vi "GPS Ublox M8N.vi"() -> (0 "Error Out":errorcluster)   [LabVIEW 2021, in "NMEA_GPS Ublox M8N.lvlib"]
uses:
  NMEA_GPS Ublox M8N.lvlib
  NMEA/NMEA_GNVTG Data.ctl
  NMEA/NMEA_Mode.ctl
  NMEA/NMEA_GNRMC Data.ctl
  NMEA/NMEA_Latitude Direction.ctl
  NMEA/NMEA_Longitude Direction.ctl
  NMEA/NMEA_GNGGA Data.ctl
  NMEA/NMEA_GPS Quality.ctl
  NMEA/NMEA_Type.ctl
  D:/My Projects/GitHub/3. GMap 1.7.0/Data/GMap.NET.WindowsForms.dll
  Data/GMap.NET.WindowsForms.dll
  Map Functions/ctlSeqFNs.ctl
  Map Functions/ctlInput4PtsColl.ctl
  fbf526f2-a788-4282-be0c-3f4d0c04ab2b.vi
  6f17bc59-fa4d-4478-9a37-96364ebc542e.vi
  Map Functions/Global Var.vi
  <vilib>/Instr/_visa.llb/VISA Configure Serial Port (Instr).vi
  <vilib>/Utility/file.llb/Write Delimited Spreadsheet (string).vi
  D:/My Projects/GitHub/3. GMap 1.7.0/Data/GMap.NET.Core.dll
  Data/GMap.NET.Core.dll
panel:
  out "MouseLng":dbl caption="Lng" format="%#.6f"
  out "MouseLat":dbl caption="Lat" format="%#.6f"
  in  "Mode":T1(ring)=enum."ServerAndCache"
  in  "Map Providers":string(combo)="27"
  in  "Zoom":dbl(slide)=14.0 min=1.0 max=20.0 step=1.0 scale=0.0..20.0
  in  "Zoom & Center":bool caption="btnZoom & Center"
  in  "Add Marker":bool
  out "Map Error":errorcluster
  in  "Error In 2":errorcluster
  in  "Marker Tooltip":enum16{"On Mouse Move", "Never", "Always"}(ring)=enum."Always"
  in  "Marker ToolTip":string="You Are Here..."
  in  "dotNetGMap":refnum<k24>(container)
  in  "Stop":bool
  in  "Serial Settings":T2={"Baud Rate"=38400, "Data Bits"=8, "Parity"=enum."None", "Stop Bits"=10, "Flow Control"=0} {"Flow Control" items=["None"=0, "XON/XOFF"=1, "RTS/CTS"=2, "DTR/DSR"=4]; "Stop Bits" items=["1.0"=10, "1.5"=15, "2.0"=20]; "Data Bits" min=5 max=8 step=1; "Baud Rate" items=["75"=75, "110"=110, "134"=134, "150"=150, "300"=300, "600"=600, "1200"=1200, "1800"=1800, "2400"=2400, "4800"=4800, "7200"=7200, "9600"=9600, "14400"=14400, "19200"=19200, "28800"=28800, "38400"=38400, "56000"=56000, "57600"=57600, "115200"=115200, "128000"=128000, "230400"=230400]}
  out "Read Data":string
  in  "COM Port":refnum<visa-resource-name>="COM18"
  in  "Timeout (ms)":u32=10000
  in  "End read on Termination Character?":bool=TRUE
  in  "Termination Char (0xA = '\\n' = LF)":u8=10 format="%.0x"
  in  "XON Character":u8=17 format="%.0x"
  in  "XOFF Character":u8=19 format="%.0x"
  in  "Input Buffer Size":u32=4096
  in  "Bytes to Read":u32=1000
  out "Actual Bytes Read":u32
  out "MessageType":T3
  in  "Error In":errorcluster
  out "$GNGGA Message":T4={"TimeStamp"=timestamp(0 s since 1904-01-01), "Latitude"=0.0, "Latitude Direction"=enum."", "Longitude"=1.0, "Longitude Direction"=enum."", "GPS Quality"=enum."GPS fix (SPS)", "Number of Satellites"=0, "Horizontal Dilution of Precision"=0.0, "Altitude above Mean-Sea-Level"=0.0, "Geoidal Separation"=0.0, "Time Since Last DGPS Update"=0.0, "DGPS Reference Station ID"=0} {"Time Since Last DGPS Update" format="%.02f [s]"; "Geoidal Separation" format="%.02f [m]"; "Altitude above Mean-Sea-Level" format="%.02f [m]"; "Horizontal Dilution of Precision" format="%.02f [HDOP]"; "Longitude" format="%0.4f [long]"; "Latitude" format="%.04f [lat]"; "TimeStamp" format="%<%.2X>T"}
  out "Latitude":dbl format="%.6f"
  out "Longitude":dbl format="%.6f"
  out "Data":string[][](table)
  out "$GNRMC Message":T8={"TimeStamp"=timestamp(0 s since 1904-01-01), "Validity"=FALSE, "Latitude"=0.0, "Latitude Direction"=enum."North", "Longitude"=0.0, "Longitude Direction"=enum."East", "Speed in Knots"=0.0, "True Course"=0.0, "Date Stamp"=timestamp(0 s since 1904-01-01), "Magnetic Variation (East/West)"=0.0} {"Magnetic Variation (East/West)" format="%.02f [deg]"; "Date Stamp" format="%<%x>T"; "True Course" format="%.02f [deg]"; "Speed in Knots" format="%.02f [kts]"; "Longitude" format="%0.4f [long]"; "Latitude" format="%.04f [lat]"; "TimeStamp" format="%<%.2X>T"}
  out "$GNVTG Message":T9={"True Course over Ground"=0.0, "Magnetic Course over Ground"=0.0, "Speed over Ground in knots"=0.0, "Speed over Ground in km/h"=1.0, "Mode"=""} {"Speed over Ground in km/h" format="%.02f [km/h]"; "Speed over Ground in knots" format="%.02f [kts]"; "Magnetic Course over Ground" format="%.02f [deg]"; "True Course over Ground" format="%.02f [deg]"}
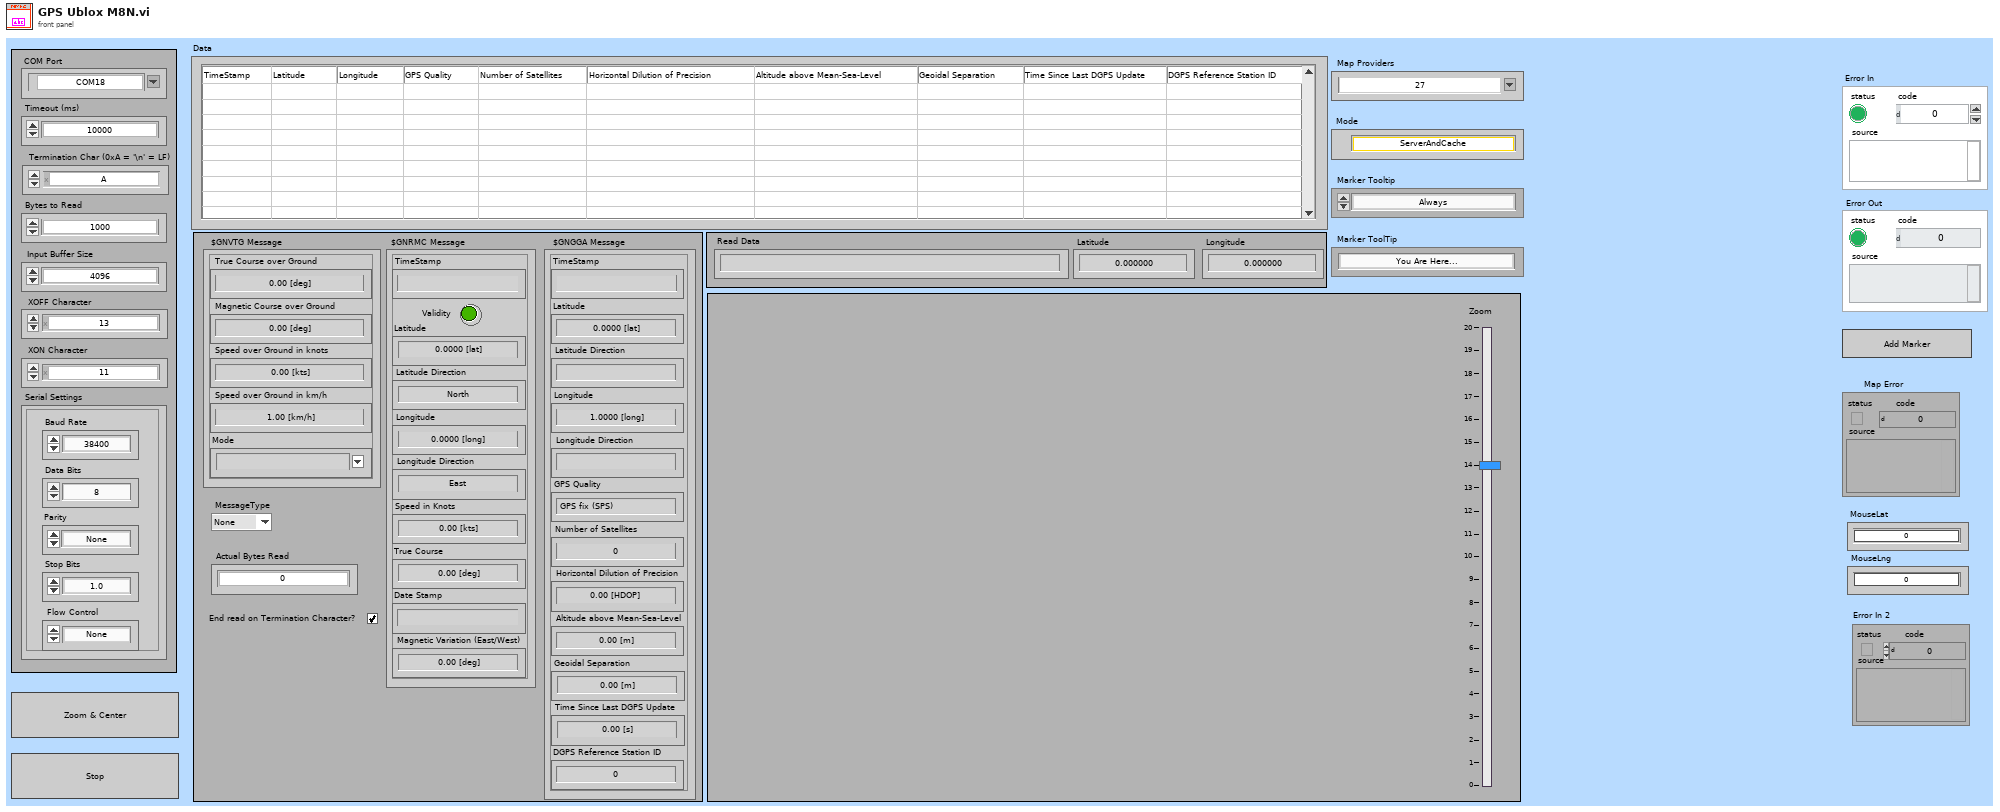
[diagram p1: front panel]
types:
  T1 = enum16{"ServerOnly", "ServerAndCache", "CacheOnly"}
  T2 = cluster{"Baud Rate":u32, "Data Bits":u16, "Parity":enum16{"None", "Odd", "Even", "Mark", "Space"}, "Stop Bits":u16, "Flow Control":u16}
  T3 = typedef "NMEA_GPS Ublox M8N.lvlib/NMEA_Type.ctl" = enum16{"None", "GGA", "VTG", "RMC"}
  T4 = typedef "NMEA_GPS Ublox M8N.lvlib/NMEA_GNGGA Data.ctl" = cluster{"TimeStamp":timestamp, "Latitude":dbl, "Latitude Direction":T5, "Longitude":dbl, "Longitude Direction":T6, "GPS Quality":T7, "Number of Satellites":i32, "Horizontal Dilution of Precision":dbl, "Altitude above Mean-Sea-Level":dbl, "Geoidal Separation":dbl, "Time Since Last DGPS Update":dbl, "DGPS Reference Station ID":i32}
  T5 = typedef "NMEA_GPS Ublox M8N.lvlib/NMEA_Latitude Direction.ctl" = enum16{"", "North", "South"}
  T6 = typedef "NMEA_GPS Ublox M8N.lvlib/NMEA_Longitude Direction.ctl" = enum16{"", "East", "West"}
  T7 = typedef "NMEA_GPS Ublox M8N.lvlib/NMEA_GPS Quality.ctl" = enum16{"Invalid", "GPS fix (SPS)", "DGPS fix", "PPS fix", "Real Time Kinematic", "Float RTK", "estimated", "Manual input mode", "Simulation mode"}
  T8 = typedef "NMEA_GPS Ublox M8N.lvlib/NMEA_GNRMC Data.ctl" = cluster{"TimeStamp":timestamp, "Validity":bool, "Latitude":dbl, "Latitude Direction":T5, "Longitude":dbl, "Longitude Direction":T6, "Speed in Knots":dbl, "True Course":dbl, "Date Stamp":timestamp, "Magnetic Variation (East/West)":dbl}
  T9 = typedef "NMEA_GPS Ublox M8N.lvlib/NMEA_GNVTG Data.ctl" = cluster{"True Course over Ground":dbl, "Magnetic Course over Ground":dbl, "Speed over Ground in knots":dbl, "Speed over Ground in km/h":dbl, "Mode":T10}
  T10 = typedef "NMEA_GPS Ublox M8N.lvlib/NMEA_Mode.ctl" = string
  T11 = typedef "NMEA_GPS Ublox M8N.lvlib/ctlSeqFNs.ctl" = enum16{"Pre - Initialize 0", "Pre - Initialize 1", "Pre - Initialize 2", "Pre - Initialize 3", "Idle", "Set Provider", "Set Scale", "Add Overlay", "Points - Create List (Container)", "Map - Marker Add Or Rmv", "Map - Markers Autofit", "Map - Markers Clear", "Error", "Exit"}
  T12 = enum32{"Invalid", "Standard", "Closed", "Hidden", "Minimized", "Maximized"}
  T13 = cluster{"Idx|Addr|City|Prov|Lng|Lat|Checked":string[], "tbCtlGUI":refnum<vi>, "PinDropLatDblClck":refnum<vi>, "PinDropLngDblClck":refnum<vi>, "MouseLat":refnum<vi>, "MouseLng":refnum<vi>, "RefScale":refnum<vi>, "RefcmbProviders":refnum<vi>, "RefMode":refnum<vi>, "EvntRefGMap":refnum<k27>, "arrRefProviders":refnum<k24>[], "arrProviderNms":string[], "dotNetGMap":refnum<k24>, "PathCurr":path, "VIRef":refnum<vi>, "arrOverlayNames":string[], "arrOverlayRefs":refnum<k24>[], "RefPointsCollPoly":refnum<k24>, "arrLatLngDF":dbl[][][], "arrLatLngPoly":dbl[][], "arrPointKeyWordOrID":string[], "MouseLatDblClck":refnum<vi>, "MouseLngDblClck":refnum<vi>}
  T14 = typedef "NMEA_GPS Ublox M8N.lvlib/ctlInput4PtsColl.ctl" = cluster{"arrLatLngActv":dbl[][], "ptKeyorID":string[], "Add":bool}
  T15 = enum16{"none", "arrow", "blue", "blue_small", "blue_dot", "blue_pushpin", "brown_small", "gray_small", "green", "green_small", "green_dot", "green_pushpin", "green_big_go", "yellow", "yellow_small", "yellow_dot", "yellow_big_pause", "yellow_pushpin", "lightblue", "lightblue_dot", "lightblue_pushpin", "orange", "orange_small", "orange_dot", "pink", "pink_dot", "pink_pushpin", "purple", "purple_small", "purple_dot", "purple_pushpin", "red", "red_small", "red_dot", "red_pushpin", "red_big_stop", "black_small", "white_small"}
  T16 = cluster{"arrOverlayRefs":refnum<k24>[], "RefPointsColl in":refnum<k24>, "arrPointKeyWordOrID":string[], "PtLatLn+KywrdOrID":T14, "arrLatLngActv":dbl[][]}
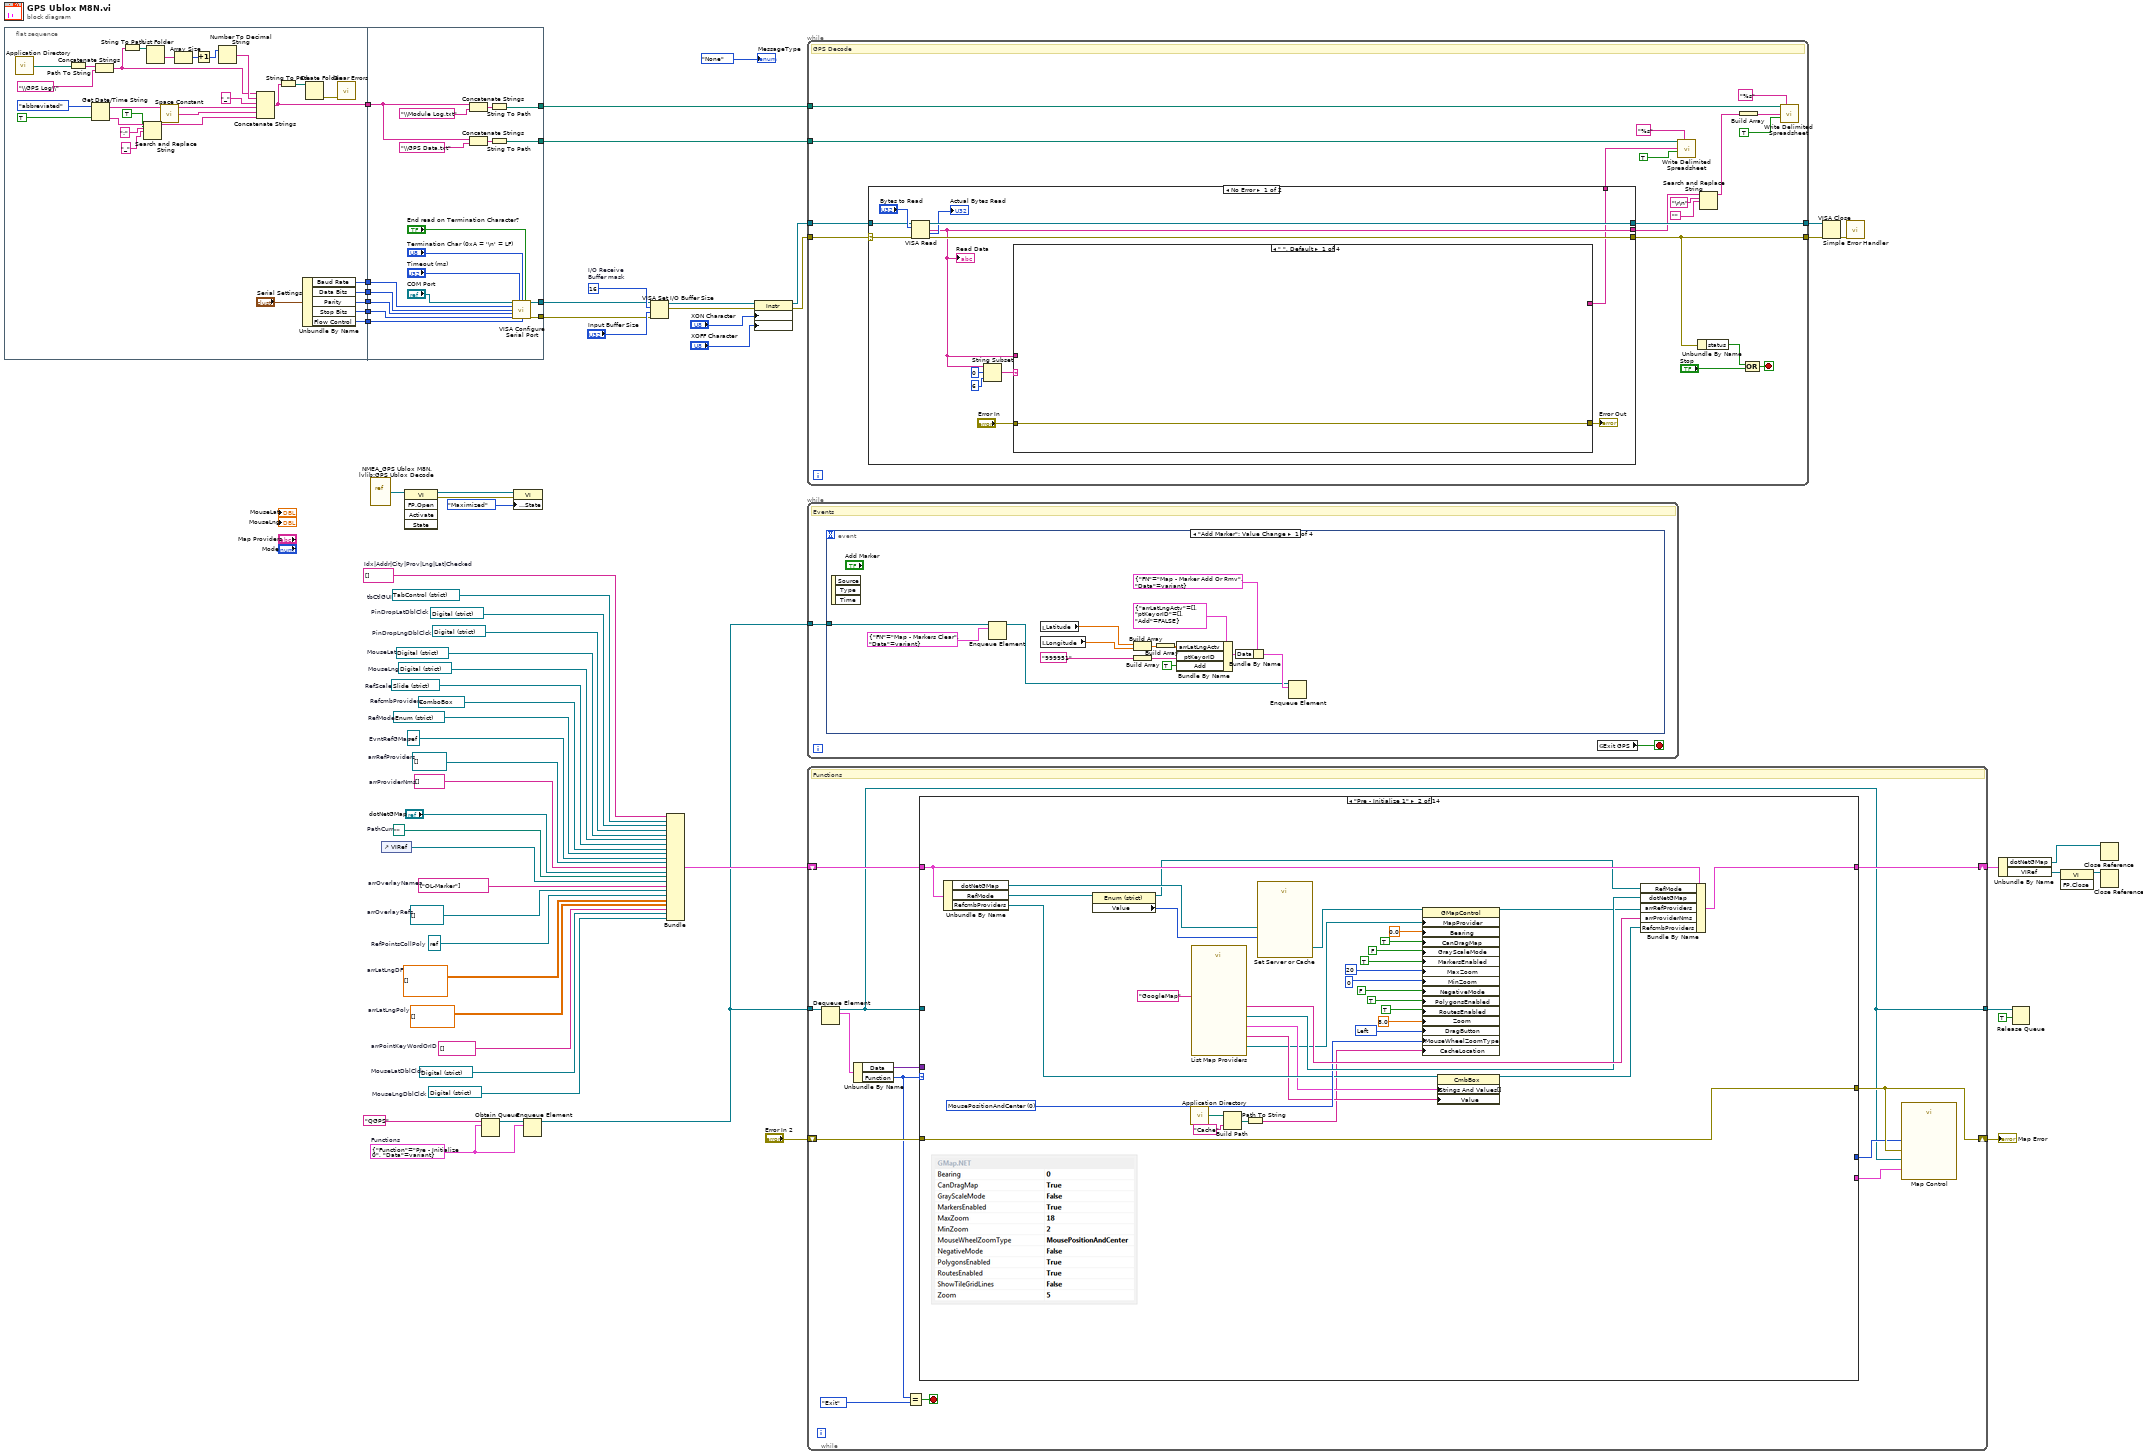
[diagram p0: block diagram]
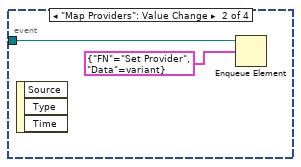
[diagram p2: hidden frame]
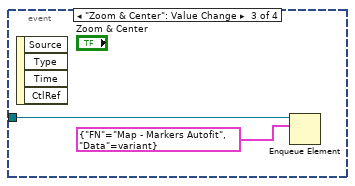
[diagram p3: hidden frame]
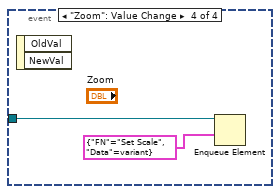
[diagram p4: hidden frame]
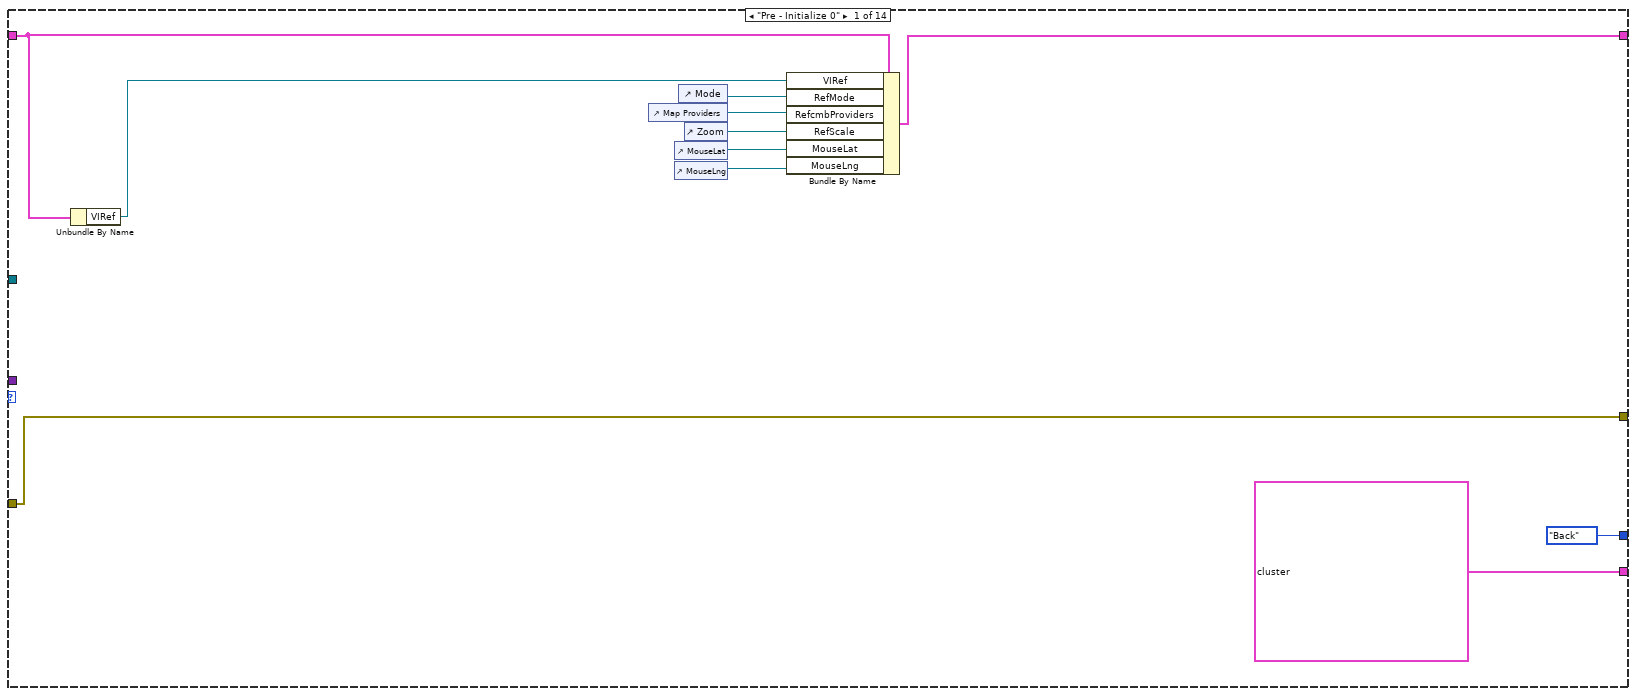
[diagram p5: hidden frame]
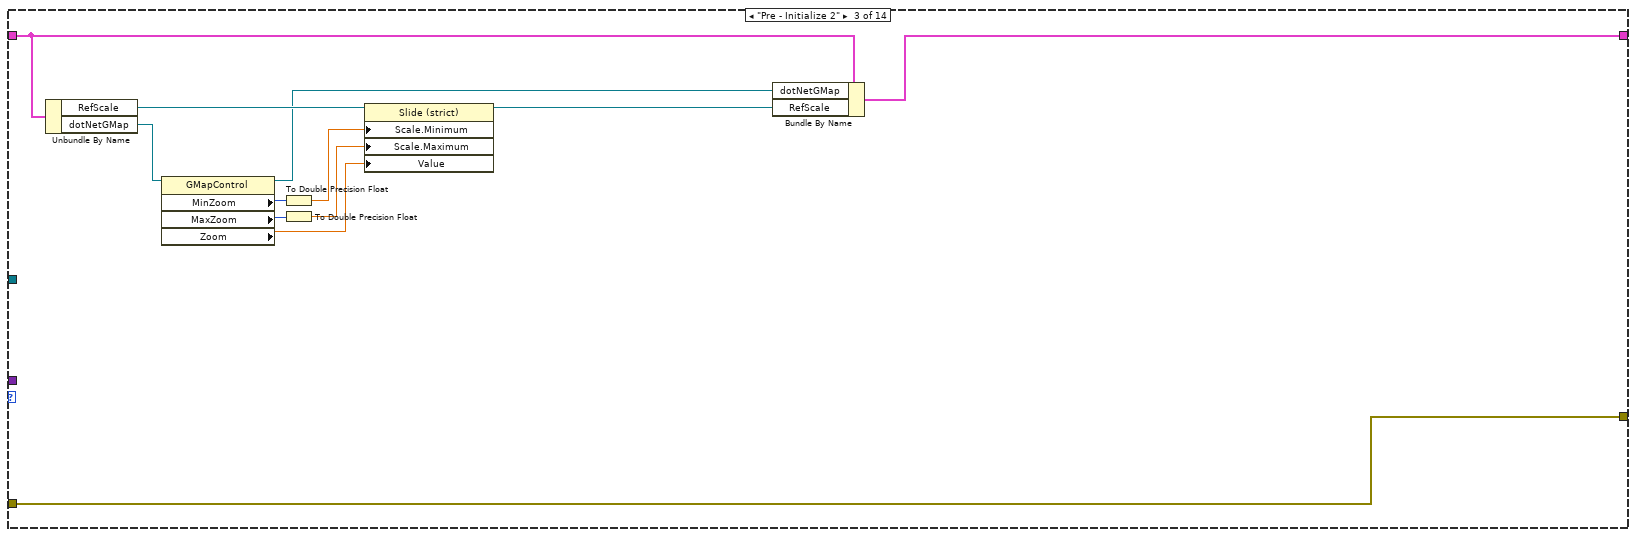
[diagram p6: hidden frame]
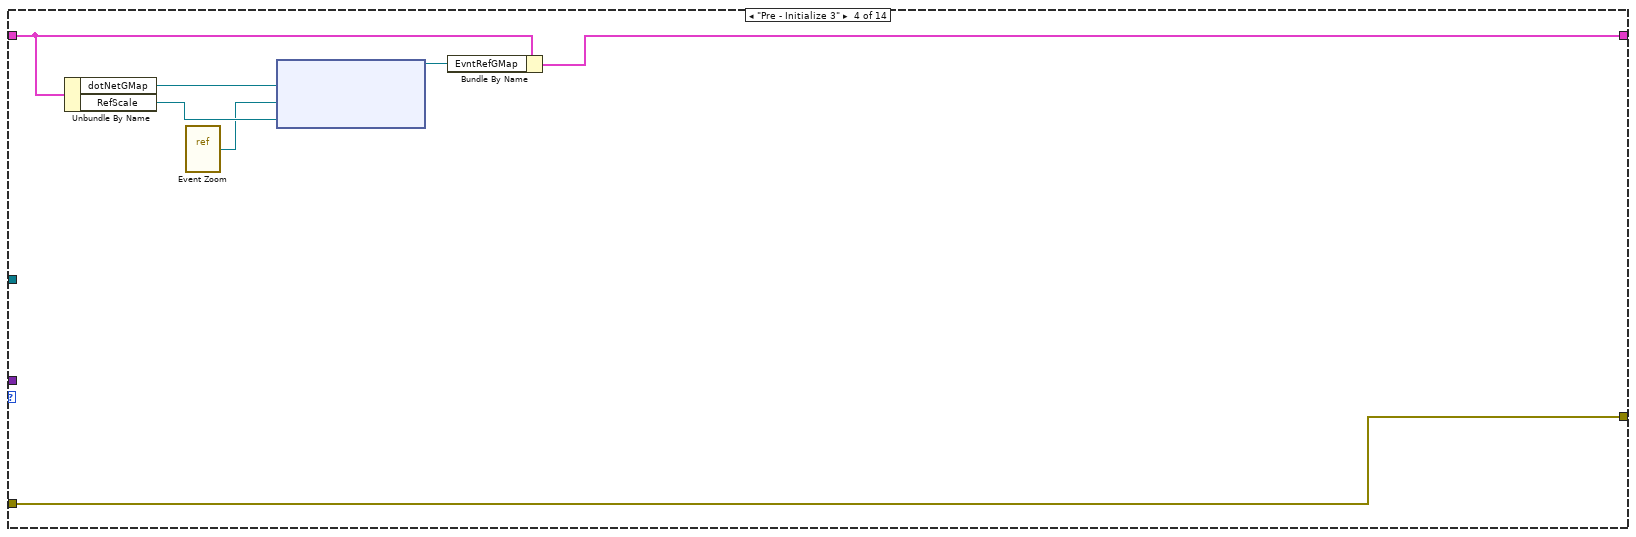
[diagram p7: hidden frame]
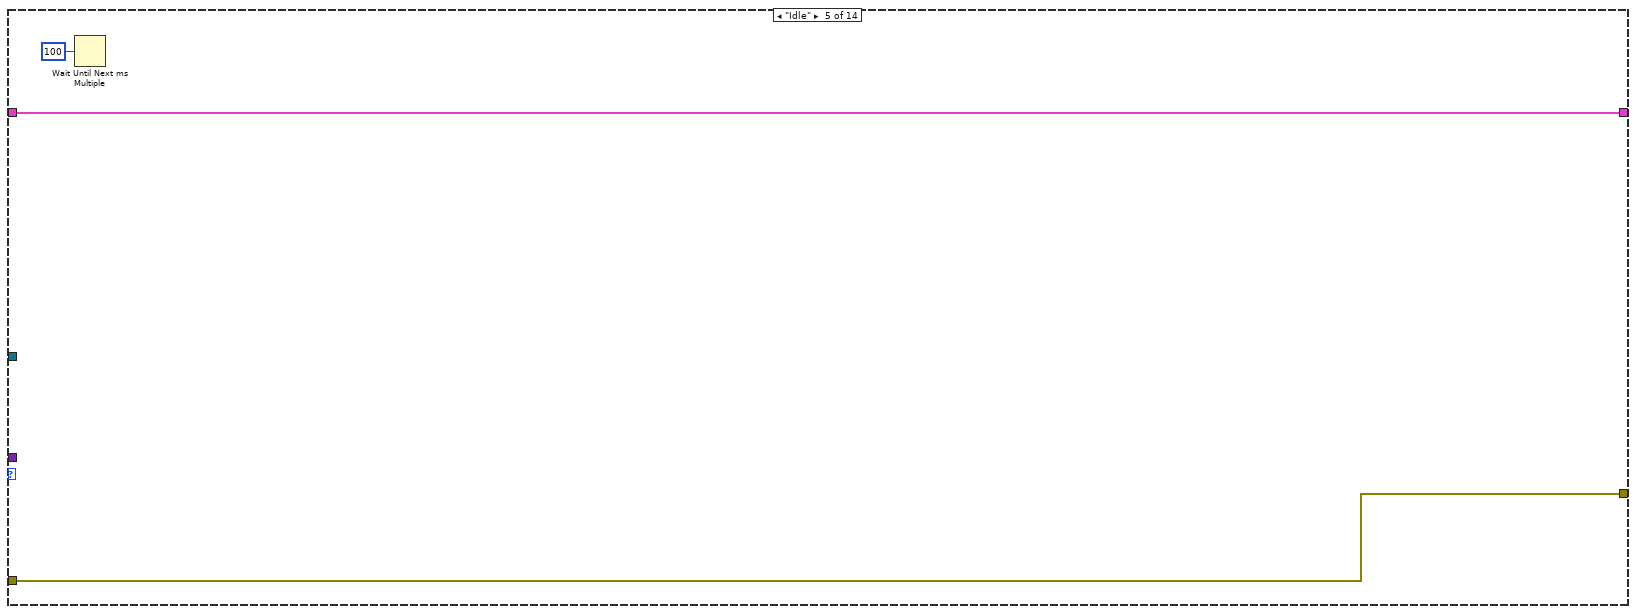
[diagram p8: hidden frame]
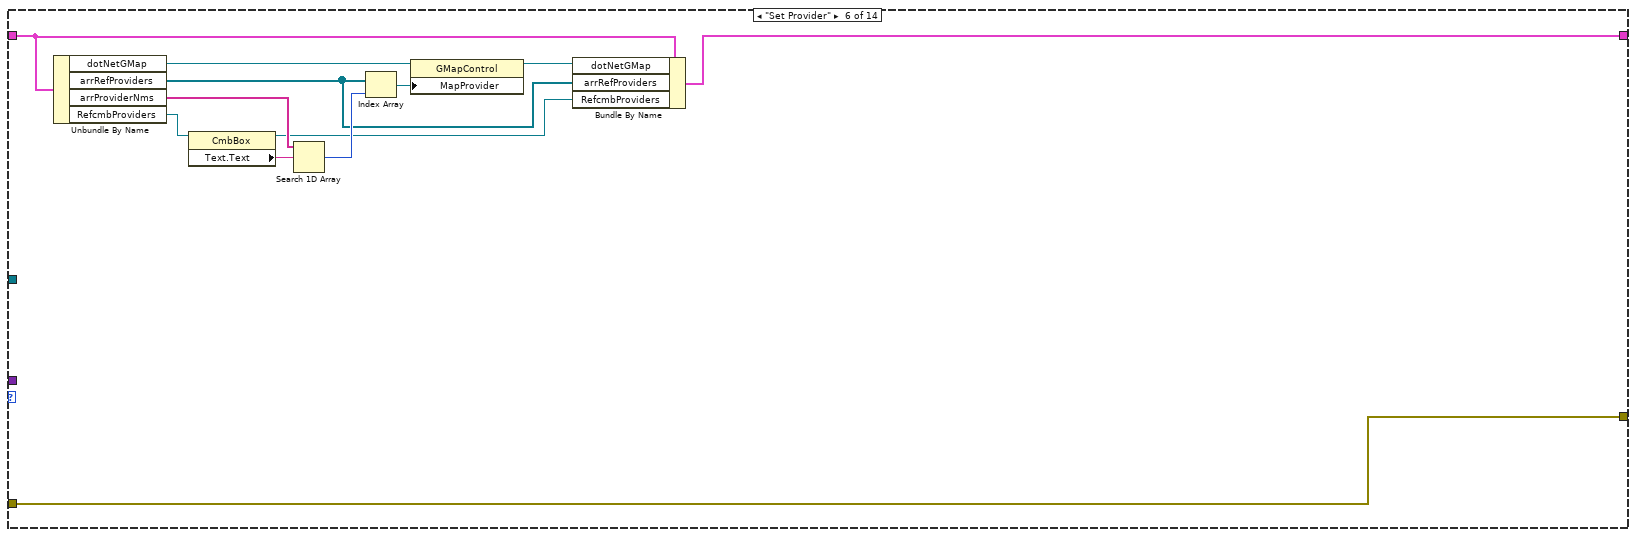
[diagram p9: hidden frame]
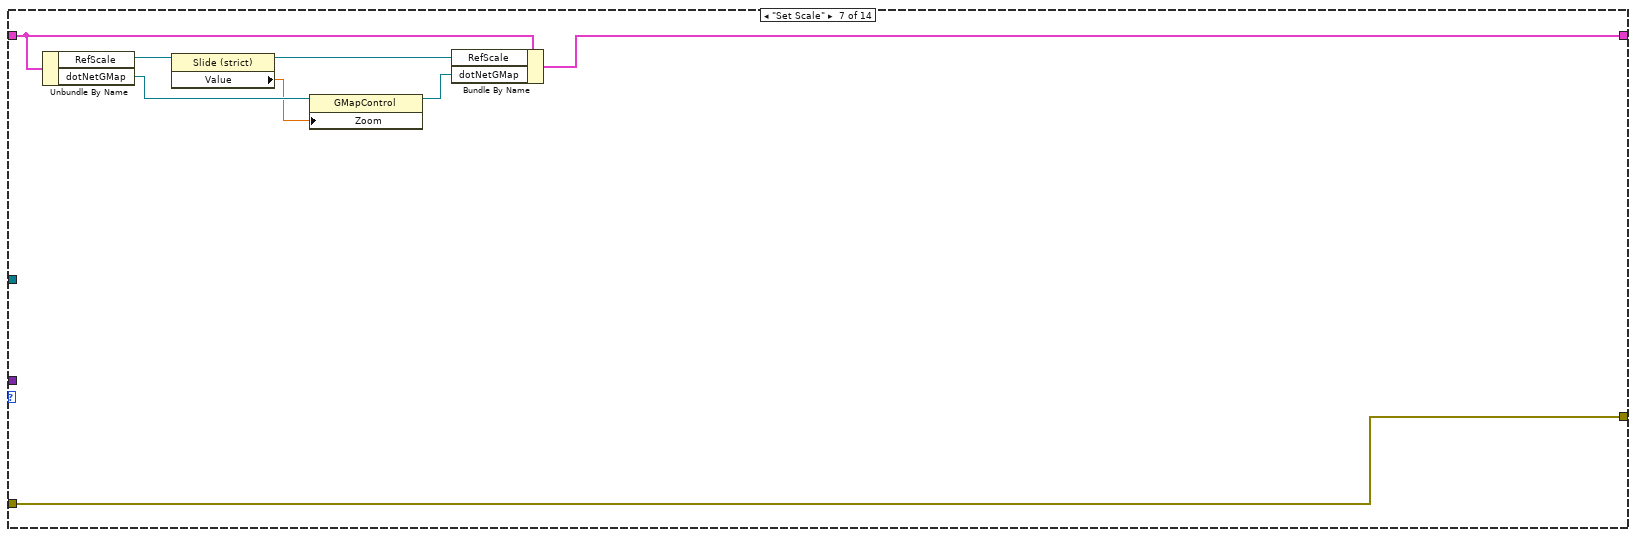
[diagram p10: hidden frame]
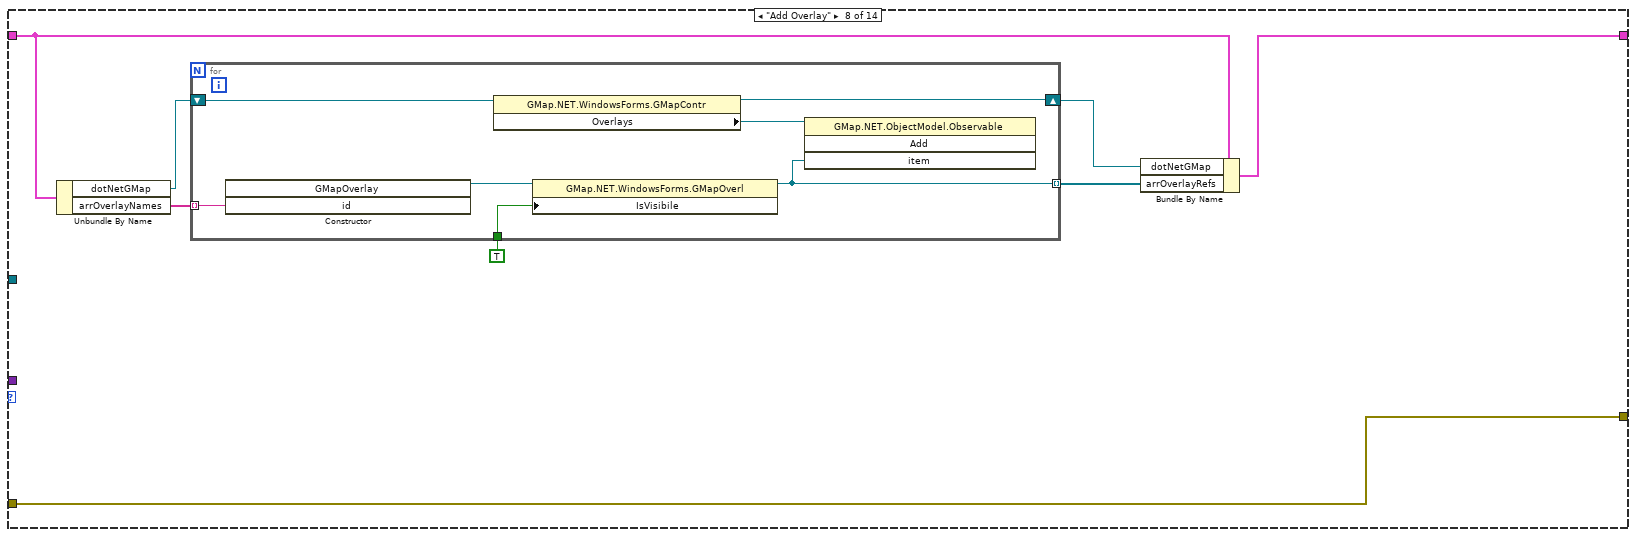
[diagram p11: hidden frame]
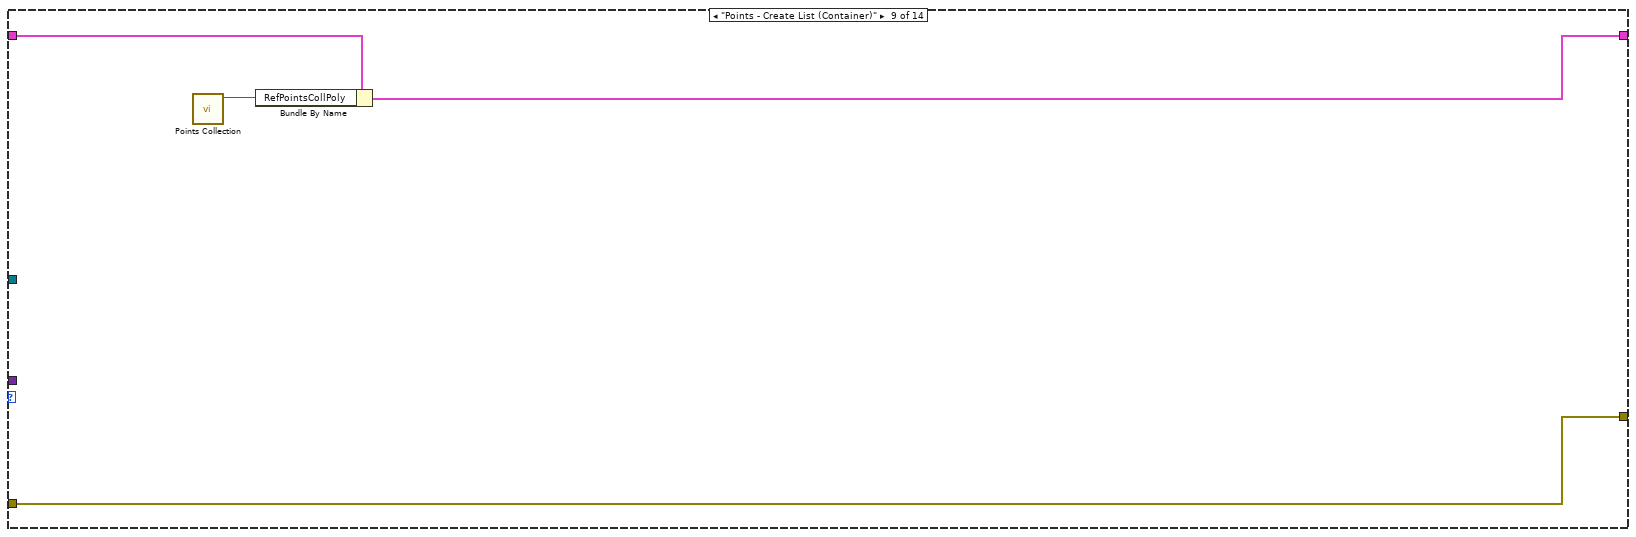
[diagram p12: hidden frame]
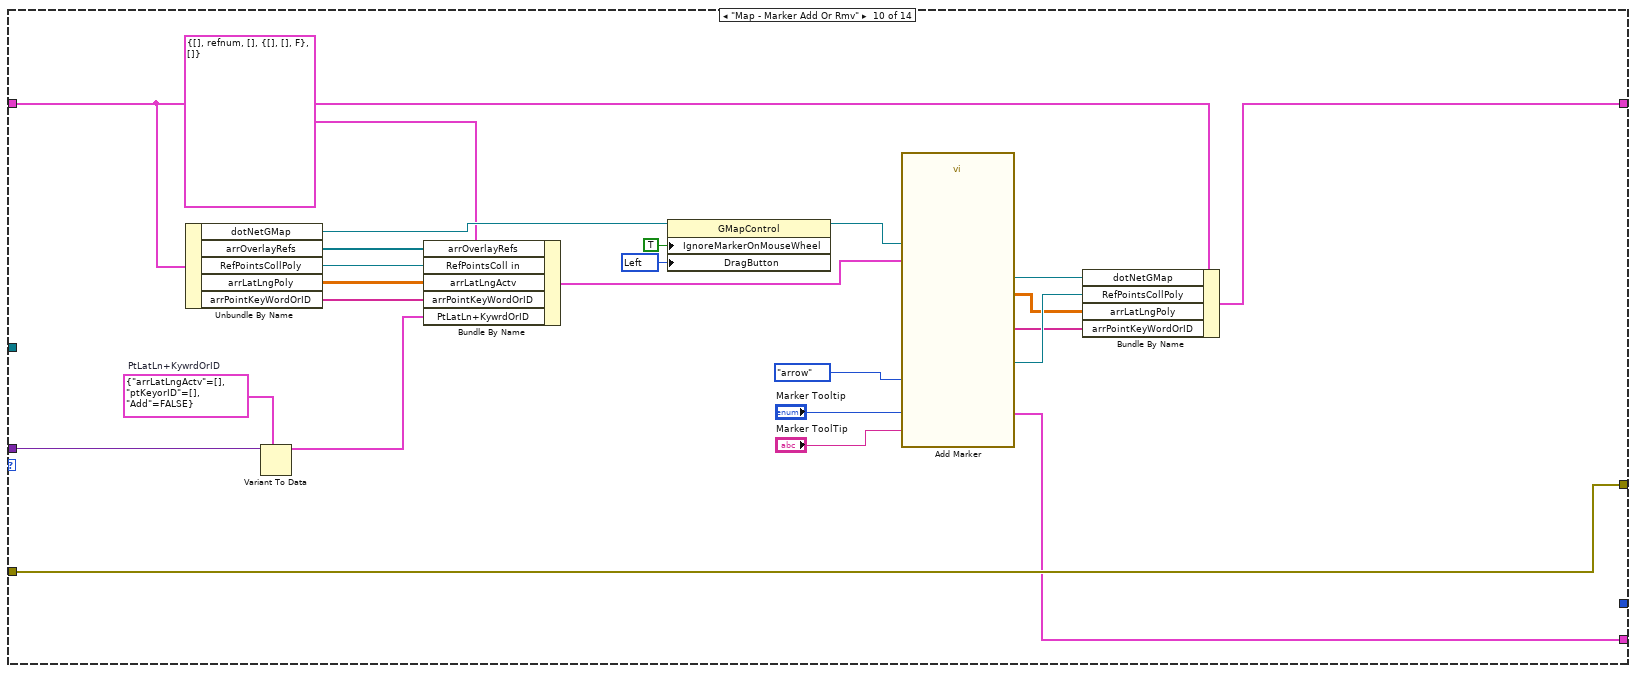
[diagram p13: hidden frame]
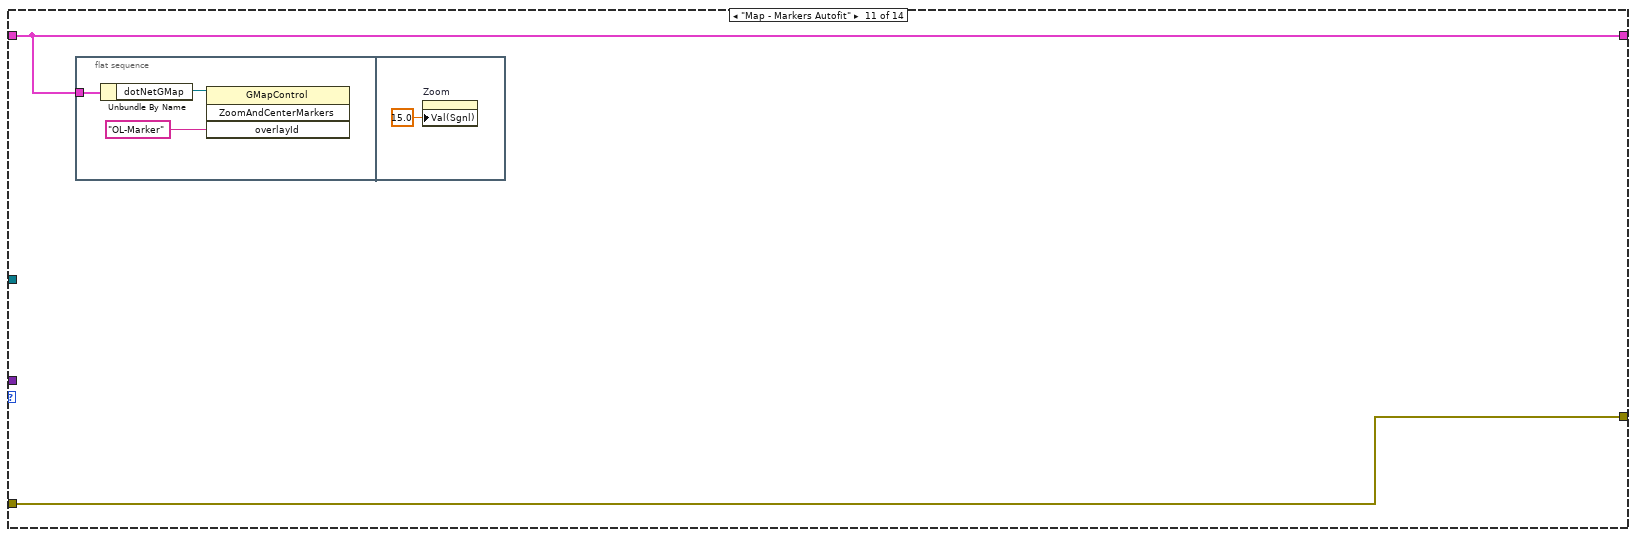
[diagram p14: hidden frame]
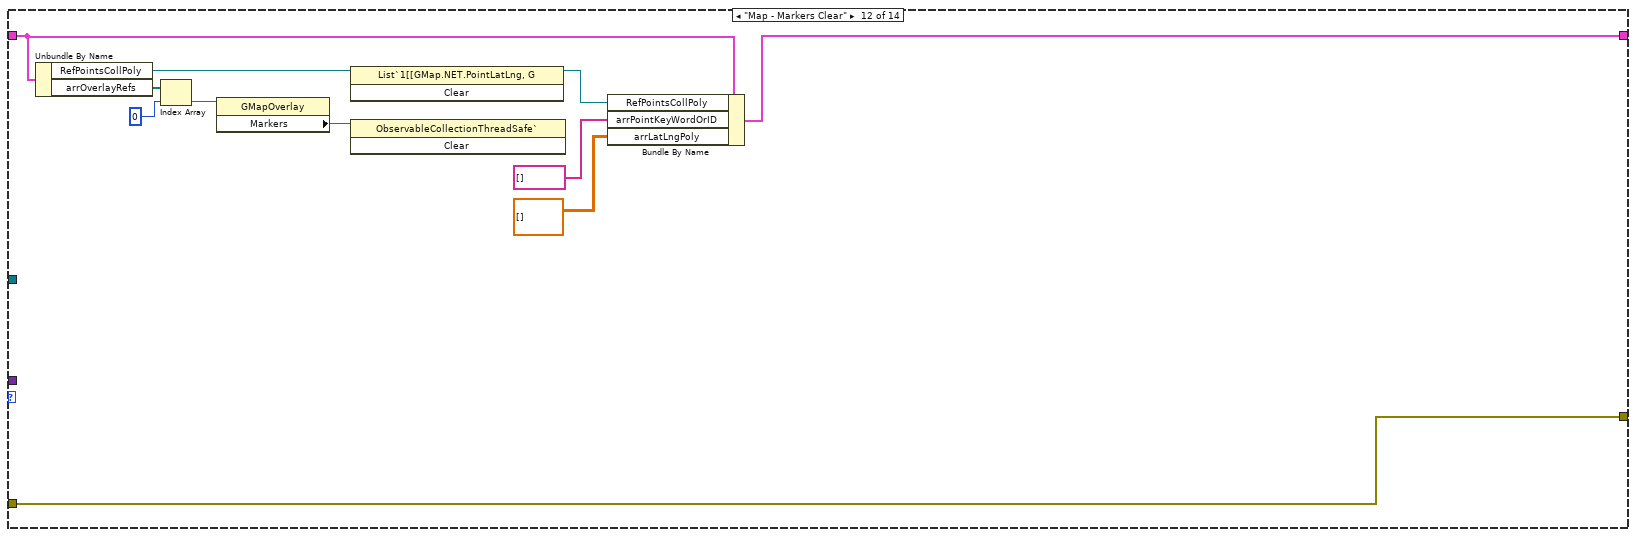
[diagram p15: hidden frame]
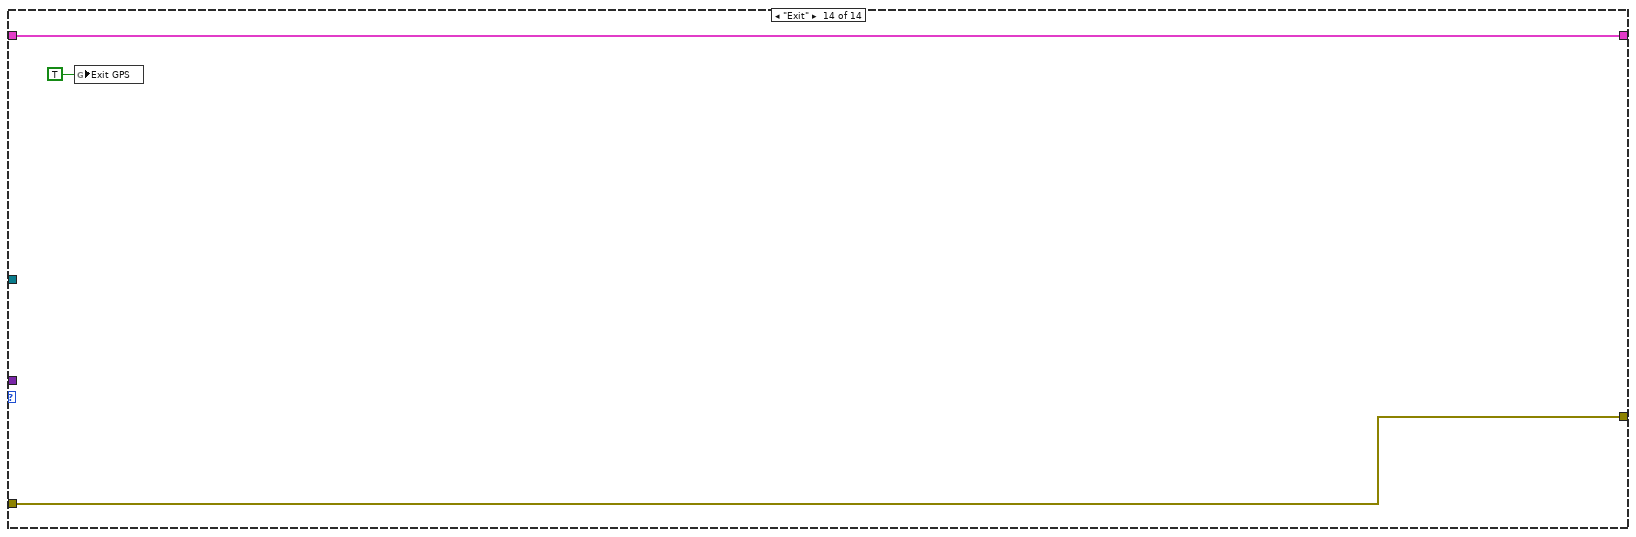
[diagram p17: hidden frame]
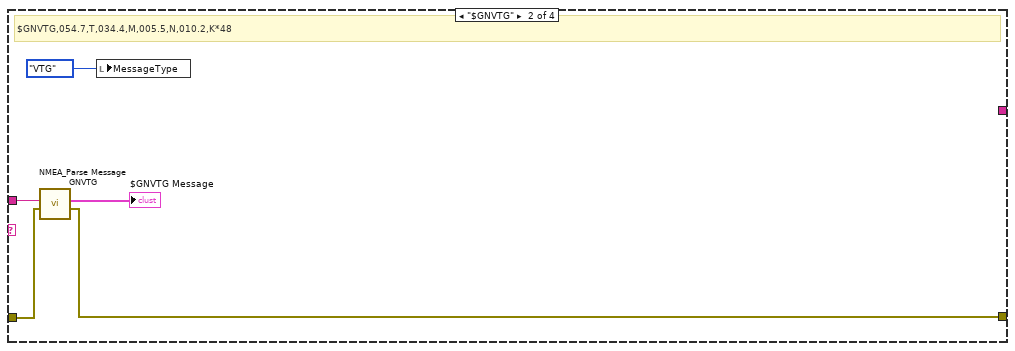
[diagram p18: hidden frame]
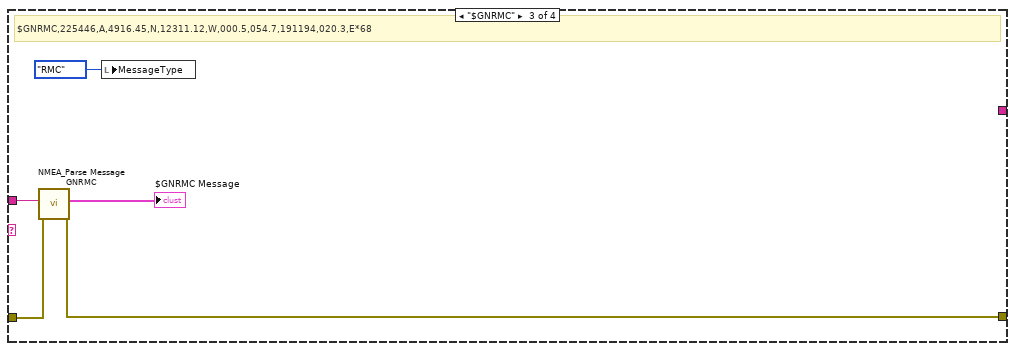
[diagram p19: hidden frame]
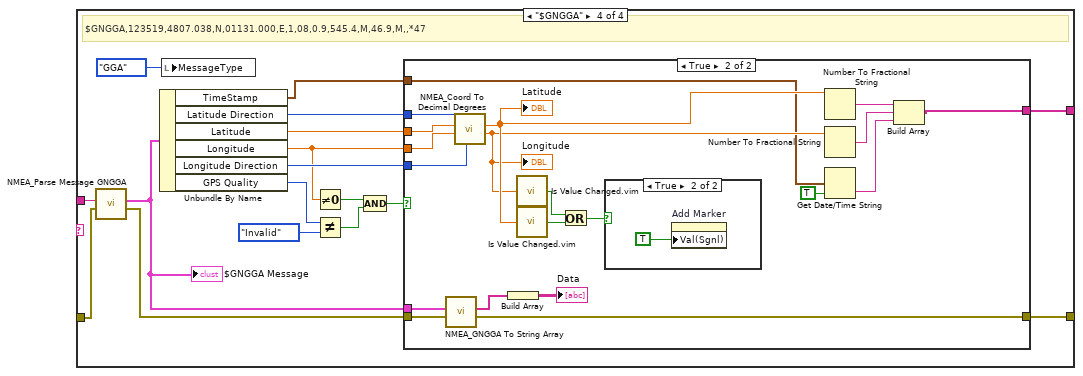
[diagram p20: hidden frame]
diagram:
  w5 = cluster{"Function":T11, "Data":variant} {"Function"=enum."Pre - Initialize 0", "Data"=variant}  # Functions
  w3 = dbl[][] []  # arrLatLngPoly
  w4 = refnum<k24> refnum  # RefPointsCollPoly
  w11 = string[] []  # Idx|Addr|City|Prov|Lng|Lat|Checked
  w12 = refnum<vi> refnum  # tbCtlGUI
  w14 = refnum<vi> refnum  # PinDropLngDblClck
  w13 = refnum<vi> refnum  # PinDropLatDblClck
  w15 = refnum<vi> refnum  # MouseLngDblClck
  w16 = refnum<vi> refnum  # MouseLatDblClck
  w17 = string[] []  # arrPointKeyWordOrID
  w18 = dbl[][][] []  # arrLatLngDF
  w19 = refnum<k24>[] []  # arrOverlayRefs
  w20 = string[] ["OL-Marker"]  # arrOverlayNames
  w21 = refnum<vi> refnum  # MouseLat
  w22 = refnum<vi> refnum  # MouseLng
  w23 = refnum<vi> refnum  # RefScale
  w26 = refnum<vi> refnum  # RefcmbProviders
  w25 = refnum<vi> refnum  # RefMode
  w27 = refnum<k27> refnum  # EvntRefGMap
  w29 = string[] []  # arrProviderNms
  w28 = refnum<k24>[] []  # arrRefProviders
  w39 = path ""  # PathCurr
  w61 = u16 16  # I/O Receive Buffer mask
  n1 = flat-sequence {
    tunnel: [w89] -> w49
    tunnel: [w88] -> w48
    tunnel: [w87] -> w47
    tunnel: [w86] -> w46
    tunnel: [w85] -> w45
    tunnel: [w64] -> w1
    tunnel: [w104] -> w51
    tunnel: [w103] -> w50
    tunnel: w49 -> [w102]
    tunnel: w48 -> [w101]
    tunnel: w47 -> [w100]
    tunnel: w46 -> [w99]
    tunnel: w45 -> [w98]
    tunnel: [w92] -> w43
    tunnel: [w91] -> w2
    tunnel: w1 -> [w94]
    frame #0 {
      n2 = call <vilib>:"Application Directory.vi"() -> ("Application Directory"=w84:path)
      n3 = Path To String(path=w84) -> (string=w77:string)
      n4 = Get Date/Time String(date format (0)=enum16{"short", "long", "abbreviated"}."abbreviated", want seconds? (F)=TRUE) -> (date string=w74:string, time string=w73:string)  [unwired: 1 in]
      n5 = Concatenate Strings(w77, "\\GPS Log\\" ("string")) -> (w82:string)
      n6 = String To Path(string=w82) -> (path=w78:path)
      n7 = Search and Replace String(replace all?=TRUE ("replace all? (F)"), input string=w73, search string=":" ("replace string (\"\")"), replace string="_" ("replace string (\"\")")) -> (result string=w76:string)  [unwired: 4 in, 3 out]
      n8 = List Folder(path=w78) -> (folder names=w79:string[])  [unwired: 3 in, 3 out]
      n9 = call <vilib>:"Space Constant.vi"() -> ("String"=w75:string)
      n10 = Array Size(array=w79) -> (size(s)=w80:i32)
      n11 = Increment(x=w80) -> (x+1=w81:i32)
      n12 = Number To Decimal String(number=w81) -> (decimal integer string=w83:string)  [unwired: 1 in]
      n13 = Concatenate Strings(w82, w83, "_" ("replace string (\"\")"), w74, w75, w76) -> (w64:string)
      n14 = String To Path(string=w64) -> (path=w63:path)
      n15 = Unbundle By Name("Serial Settings") -> ("Baud Rate"=w89:u32, "Data Bits"=w88:u16, "Parity"=w87:enum16{"None", "Odd", "Even", "Mark", "Space"}, "Stop Bits"=w86:u16, "Flow Control"=w85:u16)
      n16 = Create Folder(path (use dialog)=w63) -> (error out=w65:errorcluster)  [unwired: 2 in, 2 out]
      n17 = call <vilib>:"Clear Errors.vi"("error in (no error)"=w65) -> ()  [unwired: 5 in, 2 out]
    }
    frame #1 {
      n18 = Concatenate Strings(w94, "\\Module Log.txt" ("string")) -> (w95:string)
      n19 = Concatenate Strings(w94, "\\GPS Data.txt" ("string")) -> (w97:string)
      n20 = String To Path(string=w95) -> (path=w92:path)
      n21 = String To Path(string=w97) -> (path=w91:path)
      n22 = call-poly "VISA Configure Serial Port"("VISA resource name"="COM Port", "timeout (10sec)"="Timeout (ms)", "termination char\n(0xA = '\\n' = LF)"="Termination Char (0xA = '\\n' = LF)", "Enable Termination\nChar (T)"="End read on Termination Character?", "baud rate (9600)"=w102, "data bits (8)"=w101, "parity (0:none)"=w100, "stop bits (10: 1 bit)"=w99, "flow control (0:none)"=w98) -> ("VISA resource name out"=w104:refnum<visa-resource-name>, "error out"=w103:errorcluster)  [unwired: 1 in, 4 out]
    }
  }
  n23 = vi-ref "NMEA_GPS Ublox M8N.lvlib:GPS Ublox Decode.vi"() -> (w6:refnum<vi>)
  n24 = control-ref of="VIRef"() -> (w35:refnum<vi>)
  n25 = invoke class="VI" method="FP.Open"(reference=w6) -> (reference out=w8:refnum<vi>, error out=w7:errorcluster)  [unwired: 4 in, 3 out]
  n26 = Obtain Queue(name (unnamed)="QGPS", element data type=w5) -> (queue out=w32:refnum<queue>)  [unwired: 3 in, 2 out]
  n27 = property class="VI"(reference=w8, error in=w7, "Front Panel Window:State"=T12."Maximized") -> ()  [unwired: 2 out]
  n28 = Enqueue Element(queue=w32, element=w5) -> (queue out=w24:refnum<queue>)  [unwired: 2 in, 2 out]
  n29 = VISA Set I/O Buffer Size(VISA resource name=w51, mask (16)=w61, size (4096)="Input Buffer Size", error in (no error)=w50) -> (VISA resource name out=w59:refnum<visa-resource-name>, error out=w58:errorcluster)
  n30 = Bundle("Idx|Addr|City|Prov|Lng|Lat|Checked"=w11, "tbCtlGUI"=w12, "PinDropLatDblClck"=w13, "PinDropLngDblClck"=w14, "MouseLat"=w21, "MouseLng"=w22, "RefScale"=w23, "RefcmbProviders"=w26, "RefMode"=w25, "EvntRefGMap"=w27, "arrRefProviders"=w28, "arrProviderNms"=w29, "dotNetGMap"="dotNetGMap", "PathCurr"=w39, "VIRef"=w35, "arrOverlayNames"=w20, "arrOverlayRefs"=w19, "RefPointsCollPoly"=w4, "arrLatLngDF"=w18, "arrLatLngPoly"=w3, "arrPointKeyWordOrID"=w17, "MouseLatDblClck"=w16, "MouseLngDblClck"=w15) -> (w41:T13)  [unwired: 1 in]
  n31 = property class="Instr"(reference=w59, error in=w58, "Serial Settings:Flow Control XON Character"="XON Character", "Serial Settings:Flow Control XOFF Character"="XOFF Character") -> (reference out=w54:refnum<visa-resource-name>, error out=w55:errorcluster)
  n32 = while {
    tunnel: w55 -> [w125]
    tunnel: w54 -> [w124]
    tunnel: [w127] -> w53
    tunnel: [w126] -> w52
    tunnel: w43 -> [w120]
    tunnel: w2 -> [w115]
    stop <- w123 stop-if-true
    # "GPS Decode"
    n33 = case "Read bytes from port." shown="No Error" w125 {
      selector: w125 -> [w136 w191]
      tunnel: [w139 w191] -> w126
      tunnel: [w140 w192] -> w127
      tunnel: w124 -> [w137 w192]
      tunnel: [w130 _] -> w118
      tunnel: [w128 _] -> w114
      frame No Error {
        n34 = VISA Read(VISA resource name=w137, byte count="Bytes to Read", error in (no error)=w136) -> (VISA resource name out=w140:refnum<visa-resource-name>, read buffer=w130:string, return count=→"Actual Bytes Read":u32, error out=w139:errorcluster)
        "Read Data" <- w130
        n35 = String Subset(string=w130, offset (0)=0, length (rest)=6 ("longueur (reste)")) -> (substring=w132:string)
        n36 = case "Handling NMEA Frames" shown="\" \", Default" w132 {
          tunnel: w130 -> [_ w146 w151 w168]
          tunnel: "Error In" -> [w141 w145 w150 w156]
          tunnel: [w141 w144 w149 w155] -> w134
          tunnel: [_ _ _ w152] -> w128
          frame " ", Default {
          }
          frame "$GNVTG" {
            # "$GNVTG,054.7,T,034.4,M,005.5,N,010.2,K*48"
            n37 = call "NMEA_Parse Message GNVTG.vi"("Error In"=w145, "$GPVTG Message In"=w146) -> ("Error Out"=w144:errorcluster, "$GPVTG Message Out"=→"$GNVTG Message":T9)  [unwired: 8 in]
            n38 = local write "MessageType"(NMEA_Type."VTG" ("MessageType")) -> ()
          }
          frame "$GNRMC" {
            # "$GNRMC,225446,A,4916.45,N,12311.12,W,000.5,054.7,191194,020.3,E*68"
            n39 = call "NMEA_Parse Message GNRMC.vi"("Error In"=w150, "$GPRMC Message In"=w151) -> ("Error Out"=w149:errorcluster, "$GPRMC Message Out"=→"$GNRMC Message":T8)  [unwired: 8 in]
            n40 = local write "MessageType"(NMEA_Type."RMC" ("MessageType")) -> ()
          }
          frame "$GNGGA" {
            # "$GNGGA,123519,4807.038,N,01131.000,E,1,08,0.9,545.4,M,46.9,M,,*47"
            n41 = call "NMEA_Parse Message GNGGA.vi"("Error In"=w156, "$GPGGA Message In"=w168) -> ("Error Out"=w157:errorcluster, "$GPGGA Message Out"=w164:T4)  [unwired: 8 in]
            "$GNGGA Message" <- w164
            n42 = Unbundle By Name(w164) -> ("TimeStamp"=w153:timestamp, "Latitude Direction"=w165:T5, "Latitude"=w166:dbl, "Longitude"=w163:dbl, "Longitude Direction"=w167:T6, "GPS Quality"=w158:T7)
            n43 = local write "MessageType"(NMEA_Type."GGA" ("MessageType")) -> ()
            n44 = Not Equal To 0?(x=w163) -> (x != 0?=w161:bool)
            n45 = Not Equal?(x=w158, y=NMEA_GPS_Quality."Invalid" ("GPS-Quality")) -> (x != y?=w159:bool)
            n46 = Compound Arithmetic op=AND(w161, w159) -> (w162:bool)
            n47 = case shown="True" w162 {
              tunnel: w167 -> [_ w189]
              tunnel: w166 -> [_ w186]
              tunnel: w165 -> [_ w185]
              tunnel: w164 -> [_ w181]
              tunnel: w163 -> [_ w187]
              tunnel: w157 -> [w169 w184]
              tunnel: [w169 w183] -> w155
              tunnel: w153 -> [_ w175]
              tunnel: [_ w171] -> w152
              frame False {
              }
              frame True {
                n48 = call "NMEA_GNGGA To String Array.vi"("Error In"=w184, "$GPGGA Message In"=w181) -> ("Error Out"=w183:errorcluster, "$GPGGA Message Out"=w188:string[])  [unwired: 8 in]
                n49 = call "NMEA_Coord To Decimal Degrees.vi"("Longitude-Direction"=w189, "Latitude-Direction"=w185, "Longitude"=w187, "Latitude"=w186) -> ("Longitude"=w176:dbl, "Latitude"=w177:dbl)  [unwired: 6 in]
                "Latitude" <- w177
                "Longitude" <- w176
                n50 = Build Array(w188) -> (→"Data":string[][])
                n51 = call "Is Value Changed.vim"("value"=w176) -> ("changed or first call?"=w180:bool)
                n52 = call "Is Value Changed.vim"("value"=w177) -> ("changed or first call?"=w179:bool)
                n53 = Or(x=w180, y=w179) -> (x .or. y?=w178:bool)
                n54 = case shown="True" w178 {
                  frame False {
                  }
                  frame True {
                    n55 = property on="Add Marker" class="Bool (strict)"("Val(Sgnl)"=TRUE) -> ()  [unwired: 2 in, 2 out]
                  }
                }
                n56 = Number To Fractional String(number=w177) -> (F-format string=w174:string)  [unwired: 3 in]
                n57 = Number To Fractional String(number=w176) -> (F-format string=w173:string)  [unwired: 3 in]
                n58 = Get Date/Time String(seconds (now)=w175, want seconds? (F)=TRUE) -> (time string=w172:string)  [unwired: 1 in, 1 out]
                n59 = Build Array(w174, w173, w172) -> (w171:string[])
              }
            }
          }
        }
        "Error Out" <- w134
      }
      frame Error {
      }
    }
    n60 = call-poly <vilib>:"Write Delimited Spreadsheet.vi"("file path (dialog if empty)"=w115, "format (%s)"="%s" ("format string"), "1D data"=w114, "append to file? (new file:F)"=TRUE) -> ()  [unwired: 10 in, 2 out]
    n61 = Unbundle By Name(w126) -> ("status"=w122:bool)
    n62 = Search and Replace String(input string=w118, search string="\r\n", replace string="" ("replace string (\"\")")) -> (result string=w116:string)  [unwired: 5 in, 3 out]
    n63 = Build Array(w116) -> (w112:string[])
    n64 = Compound Arithmetic op=OR(w122, "Stop") -> (w123:bool)
    n65 = call-poly <vilib>:"Write Delimited Spreadsheet.vi"("file path (dialog if empty)"=w120, "format (%s)"="%s" ("format string"), "1D data"=w112, "append to file? (new file:F)"=TRUE) -> ()  [unwired: 10 in, 2 out]
  }
  n66 = while {
    tunnel: w24 -> [w193]
    stop <- w194 stop-if-true
    # "Events"
    n67 = event shown="[0] \"Add Marker\": Value Change" {
      selector: _ -> [_ _ _ _]
      dyn-events: _ -> [_ _ _ _]
      timeout: _ -> [_ _ _ _]
      tunnel: w193 -> [w198 w210 w212 w214]
      event "Add Marker": Value Change {
        n68 = event-data() -> ()  [unwired: 1 in, 3 out]
        n69 = Enqueue Element(queue=w198, element=cluster{"FN":T11, "Data":variant} {"FN"=enum."Map - Markers Clear", "Data"=variant}) -> (queue out=w197:refnum<queue>)  [unwired: 2 in, 2 out]
        n70 = local read "Latitude"() -> (w196:dbl)
        n71 = local read "Longitude"() -> (w195:dbl)
        n72 = Build Array(w196, w195) -> (w206:dbl[])
        n73 = Build Array("999951") -> (w203:string[])
        n74 = Build Array(w206) -> (w205:dbl[][])
        n75 = Bundle By Name(cluster=T14 {"arrLatLngActv"=[], "ptKeyorID"=[], "Add"=FALSE} ("PtLatLn+KywrdOrID"), "arrLatLngActv"=w205, "ptKeyorID"=w203, "Add"=TRUE) -> (w201:T14)
        n76 = Bundle By Name(cluster=cluster{"FN":T11, "Data":variant} {"FN"=enum."Map - Marker Add Or Rmv", "Data"=variant} ("element"), "Data"=w201) -> (w200:cluster{"FN":T11, "Data":variant})
        n77 = Enqueue Element(queue=w197, element=w200) -> ()  [unwired: 2 in, 3 out]
      }
      event "Map Providers": Value Change {
        n78 = event-data() -> ()  [unwired: 1 in, 3 out]
        n79 = Enqueue Element(queue=w210, element=cluster{"FN":T11, "Data":variant} {"FN"=enum."Set Provider", "Data"=variant}) -> ()  [unwired: 2 in, 3 out]
      }
      event "Zoom & Center": Value Change {
        n80 = event-data() -> ()  [unwired: 1 in, 4 out]
        n81 = Enqueue Element(queue=w212, element=cluster{"FN":T11, "Data":variant} {"FN"=enum."Map - Markers Autofit", "Data"=variant}) -> ()  [unwired: 2 in, 3 out]
      }
      event "Zoom": Value Change {
        n82 = event-data() -> ()  [unwired: 1 in, 2 out]
        n83 = Enqueue Element(queue=w214, element=cluster{"FN":T11, "Data":variant} {"FN"=enum."Set Scale", "Data"=variant}) -> ()  [unwired: 2 in, 3 out]
      }
    }
    n84 = global read "Global Var.vi" "Exit GPS"() -> (w194:bool)
  }
  n85 = while "FUNCTIONS" {
    shift-right: [w224] -> w38
    shift-left: "Error In 2" -> [w227]
    shift-right: [w225] -> w37
    shift-left: w41 -> [w226]
    tunnel: w24 -> [w223]
    tunnel: [w216] -> w30
    stop <- w220 stop-if-true
    # "Functions"
    n86 = Dequeue Element(queue=w223) -> (queue out=w216:refnum<queue>, element=w222:cluster{"Function":T11, "Data":variant})  [unwired: 2 in, 2 out]
    n87 = Unbundle By Name(w222) -> ("Data"=w221:variant, "Function"=w215:T11)
    n88 = Equal?(x=w215, y=ctlSeqFNs."Exit") -> (x = y?=w220:bool)
    n89 = case shown="\"Pre - Initialize 1\"" w215 {
      tunnel: w227 -> [w237 w271 w283 w290 w293 w305 w313 w321 w332 w356 w358 w373 w375 w378]
      tunnel: [w237 w271 w283 w290 w293 w305 w313 w321 w332 w356 w358 w373 w375 w378] -> w224
      tunnel: w226 -> [w236 w270 w275 w288 w292 w302 w310 w319 w330 w354 w357 w369 w374 w377]
      tunnel: [w234 w269 w272 w287 w292 w301 w308 w317 w331 w352 w357 w368 w374 w377] -> w225
      tunnel: w221 -> [_ _ _ _ _ _ _ _ _ w355 _ _ _ _]
      tunnel: [cluster{"FN":T11, "Data":variant}[] [{"FN"=enum."Pre - Initialize 1", "Data"=variant}, {"FN"=enum."Pre - Initialize 2", "Data"=variant}, {"FN"=enum."Pre - Initialize 3", "Data"=variant}, {"FN"=enum."Idle", "Data"=variant}, {"FN"=enum."Add Overlay", "Data"=variant}, {"FN"=enum."Points - Create List (Container)", "Data"=variant}, {"FN"=enum."Map - Markers Autofit", "Data"=variant}] ("QFNs") _ _ _ _ _ _ _ _ w336 _ _ _ _] -> w218
      tunnel: [enum16{"Back", "Front", "Replace"}."Back" ("Enum") _ _ _ _ _ _ _ _ _ _ _ _ _] -> w217
      tunnel: w216 -> [_ _ _ _ _ _ _ _ _ _ _ _ _ _]
      frame "Pre - Initialize 0" {
        n90 = Unbundle By Name(w236) -> ("VIRef"=w235:refnum<vi>)
        n91 = control-ref of="Map Providers"() -> (w232:refnum<vi>)
        n92 = control-ref of="MouseLat"() -> (w231:refnum<vi>)
        n93 = control-ref of="MouseLng"() -> (w230:refnum<vi>)
        n94 = control-ref of="Mode"() -> (w233:refnum<vi>)
        n95 = control-ref of="Zoom"() -> (w229:refnum<vi>)
        n96 = Bundle By Name(cluster=w236, "VIRef"=w235, "RefMode"=w233, "RefcmbProviders"=w232, "RefScale"=w229, "MouseLat"=w231, "MouseLng"=w230) -> (w234:T13)
      }
      frame "Pre - Initialize 1" {
        w247 = 1048576 items=["None"=0, "Left"=1048576, "Right"=2097152, "Middle"=4194304, "XButton1"=8388608, "XButton2"=16777216] ("DragButton")
        w259 = 0 items=["MousePositionAndCenter", "MousePositionWithoutCenter", "ViewCenter"] ("MouseWheelZoomType")
        n97 = Unbundle By Name(w270) -> ("dotNetGMap"=w261:refnum<k24>, "RefMode"=w253:refnum<vi>, "RefcmbProviders"=w251:refnum<vi>)
        n98 = property class="Enum (strict)"(reference=w253) -> (reference out=w248:refnum<vi>, "Value"=w252:T1)  [unwired: 1 in, 1 out]
        n99 = call <vilib>:"Application Directory.vi"() -> ("Application Directory"=w242:path)
        n100 = call "List Map Providers.vi"("InitProviders"="GoogleMap") -> ("IdxInitPrvd"=w246:string, "SelProvider"=w245:refnum<k24>, "cmbProviders"=w250:cluster{"Name":string, string}[], "arrRefProviders"=w267:refnum<k24>[], "arr1DProviders"=w268:string[])  [unwired: 6 in]
        n101 = Build Path(base path=w242, name or relative path="Cache") -> (appended path=w240:path)
        n102 = Path To String(path=w240) -> (string=w239:string)
        n103 = call "Set Server or Cache.vi"("Mode"=w252, ".NET Refnum in"=w261) -> (".NET Refnum out"=w260:refnum<k24>)  [unwired: 9 in]
        n104 = property class="GMapControl"(reference=w260, "MapProvider"=w245, "Bearing"=sgl 0.0, "CanDragMap"=TRUE, "GrayScaleMode"=FALSE ("CanDragMap"), "MarkersEnabled"=TRUE, "MaxZoom"=20, "MinZoom"=0, "NegativeMode"=FALSE, "PolygonsEnabled"=TRUE, "RoutesEnabled"=TRUE, "Zoom"=8.0, "DragButton"=w247, "MouseWheelZoomType"=w259, "CacheLocation"=w239) -> (reference out=w244:refnum<k24>)  [unwired: 1 in, 1 out]
        n105 = property class="CmbBox"(reference=w251, "Strings And Values[]"=w250, "Value"=w246) -> (reference out=w249:refnum<vi>)  [unwired: 1 in, 1 out]
        n106 = Bundle By Name(cluster=w270, "RefMode"=w248, "dotNetGMap"=w244, "arrRefProviders"=w267, "arrProviderNms"=w268, "RefcmbProviders"=w249) -> (w269:T13)
      }
      frame "Pre - Initialize 2" {
        n107 = Unbundle By Name(w275) -> ("RefScale"=w281:refnum<vi>, "dotNetGMap"=w282:refnum<k24>)
        n108 = property class="GMapControl"(reference=w282) -> (reference out=w273:refnum<k24>, "MinZoom"=w279:i32, "MaxZoom"=w278:i32, "Zoom"=w280:dbl)  [unwired: 1 in, 1 out]
        n109 = To Double Precision Float(number=w279) -> (double precision float=w277:dbl)
        n110 = To Double Precision Float(number=w278) -> (double precision float=w276:dbl)
        n111 = property class="Slide (strict)"(reference=w281, "Scale.Minimum"=w277, "Scale.Maximum"=w276, "Value"=w280) -> (reference out=w274:refnum<vi>)  [unwired: 1 in, 1 out]
        n112 = Bundle By Name(cluster=w275, "dotNetGMap"=w273, "RefScale"=w274) -> (w272:T13)
      }
      frame "Pre - Initialize 3" {
        n113 = Unbundle By Name(w288) -> ("dotNetGMap"=w289:refnum<k24>, "RefScale"=w285:refnum<vi>)
        n114 = vi-ref "Event Zoom.vi"() -> ("vi reference"=w284:refnum<vi>)
        n115 = node(w289, w284, w285) -> (w286:refnum<k27>)  [unwired: 2 in, 1 out]
        n116 = Bundle By Name(cluster=w288, "EvntRefGMap"=w286) -> (w287:T13)
      }
      frame "Idle" {
        n117 = Wait Until Next ms Multiple(millisecond multiple=u32 100) -> ()  [unwired: 1 out]
      }
      frame "Set Provider" {
        n118 = Unbundle By Name(w302) -> ("dotNetGMap"=w303:refnum<k24>, "arrRefProviders"=w296:refnum<k24>[], "arrProviderNms"=w299:string[], "RefcmbProviders"=w304:refnum<vi>)
        n119 = property class="CmbBox"(reference=w304) -> (reference out=w297:refnum<vi>, "Text.Text"=w300:string)  [unwired: 1 in, 1 out]
        n120 = Search 1D Array(1D array=w299, element=w300) -> (index of element=w298:i32)  [unwired: 1 in]
        n121 = Index Array(array=w296, index=w298) -> (element=w295:refnum<k24>)
        n122 = property class="GMapControl"(reference=w303, "MapProvider"=w295) -> (reference out=w294:refnum<k24>)  [unwired: 1 in, 1 out]
        n123 = Bundle By Name(cluster=w302, "dotNetGMap"=w294, "arrRefProviders"=w296, "RefcmbProviders"=w297) -> (w301:T13)
      }
      frame "Set Scale" {
        n124 = Unbundle By Name(w310) -> ("RefScale"=w311:refnum<vi>, "dotNetGMap"=w312:refnum<k24>)
        n125 = property class="Slide (strict)"(reference=w311) -> (reference out=w309:refnum<vi>, "Value"=w306:dbl)  [unwired: 1 in, 1 out]
        n126 = property class="GMapControl"(reference=w312, "Zoom"=w306) -> (reference out=w307:refnum<k24>)  [unwired: 1 in, 1 out]
        n127 = Bundle By Name(cluster=w310, "RefScale"=w309, "dotNetGMap"=w307) -> (w308:T13)
      }
      frame "Add Overlay" {
        n128 = Unbundle By Name(w319) -> ("dotNetGMap"=w316:refnum<k24>, "arrOverlayNames"=w320:string[])
        n129 = for {
          tunnel: w320 -> [w328] mode=indexing
          tunnel: [w322] -> w318 mode=indexing
          shift-right: [w325] -> w315
          shift-left: w316 -> [w327]
          tunnel: TRUE ("IsVisibile") -> [w324]
          n130 = constructor class="GMap.NET.WindowsForms.GMapOverl"("id"=w328) -> (reference out=w323:refnum<k24>)  [unwired: 3 in, 3 out]
          n131 = property class="GMap.NET.WindowsForms.GMapContr"(reference=w327) -> (reference out=w325:refnum<k24>, "Overlays"=w326:refnum<k24>)  [unwired: 1 in, 1 out]
          n132 = property class="GMap.NET.WindowsForms.GMapOverl"(reference=w323, "IsVisibile"=w324) -> (reference out=w322:refnum<k24>)  [unwired: 1 in, 1 out]
          n133 = invoke class="GMap.NET.ObjectModel.Observable" method="Add"(reference=w326, "item"=w322) -> ()  [unwired: 2 in, 4 out]
        }
        n134 = Bundle By Name(cluster=w319, "dotNetGMap"=w315, "arrOverlayRefs"=w318) -> (w317:T13)
      }
      frame "Points - Create List (Container)" {
        n135 = call "Points Collection.vi"() -> ("RefPointsColl"=w329:refnum<k24>)  [unwired: 11 in]
        n136 = Bundle By Name(cluster=w330, "RefPointsCollPoly"=w329) -> (w331:T13)
      }
      frame "Map - Marker Add Or Rmv" {
        w335 = T14 {"arrLatLngActv"=[], "ptKeyorID"=[], "Add"=FALSE}  # PtLatLn+KywrdOrID
        w339 = 1048576 items=["None"=0, "Left"=1048576, "Right"=2097152, "Middle"=4194304, "XButton1"=8388608, "XButton2"=16777216] ("DragButton")
        n137 = Unbundle By Name(w354) -> ("dotNetGMap"=w351:refnum<k24>, "arrOverlayRefs"=w347:refnum<k24>[], "RefPointsCollPoly"=w346:refnum<k24>, "arrLatLngPoly"=w345:dbl[][], "arrPointKeyWordOrID"=w344:string[])
        n138 = Variant To Data(type=w335, Variant=w355) -> (data=w342:T14)  [unwired: 1 in, 1 out]
        n139 = Bundle By Name(cluster=T16 {"arrOverlayRefs"=[], "RefPointsColl in"=refnum, "arrPointKeyWordOrID"=[], "PtLatLn+KywrdOrID"={"arrLatLngActv"=[], "ptKeyorID"=[], "Add"=FALSE}, "arrLatLngActv"=[]} ("Inputs"), "arrOverlayRefs"=w347, "RefPointsColl in"=w346, "arrLatLngActv"=w345, "arrPointKeyWordOrID"=w344, "PtLatLn+KywrdOrID"=w342) -> (w343:T16)
        n140 = property class="GMapControl"(reference=w351, "IgnoreMarkerOnMouseWheel"=TRUE, "DragButton"=w339) -> (reference out=w341:refnum<k24>)  [unwired: 1 in, 1 out]
        n141 = call "Add Marker.vi"(".NET Refnum In"=w341, "Inputs"=w343, "ToolTip Text"="Marker ToolTip", "Marker Tooltip"="Marker Tooltip", "Marker Type"=T15."arrow") -> (".NET Refnum Out"=w338:refnum<k24>, "RefPointsColl - Out"=w353:refnum<k24>, "arrPtKyOrId"=w349:string[], "arrLat|LngActv"=w350:dbl[][], "QFNs"=w336:cluster{"FN":T11, "Data":variant}[])  [unwired: 8 in, 2 out]
        n142 = Bundle By Name(cluster=w354, "dotNetGMap"=w338, "RefPointsCollPoly"=w353, "arrLatLngPoly"=w350, "arrPointKeyWordOrID"=w349) -> (w352:T13)
      }
      frame "Map - Markers Autofit" {
        n143 = flat-sequence {
          tunnel: w357 -> [w359]
          frame #0 {
            n144 = Unbundle By Name(w359) -> ("dotNetGMap"=w361:refnum<k24>)
            n145 = invoke class="GMapControl" method="ZoomAndCenterMarkers"(reference=w361, "overlayId"="OL-Marker") -> ()  [unwired: 2 in, 4 out]
          }
          frame #1 {
            n146 = property on="Zoom" class="Slide (strict)"("Val(Sgnl)"=15.0 ("Value (Signaling)")) -> ()  [unwired: 2 in, 2 out]
          }
        }
      }
      frame "Map - Markers Clear" {
        n147 = Unbundle By Name(w369) -> ("RefPointsCollPoly"=w365:refnum<k24>, "arrOverlayRefs"=w372:refnum<k24>[])
        n148 = Index Array(array=w372, index=0) -> (element=w371:refnum<k24>)
        n149 = property class="GMapOverlay"(reference=w371) -> ("Markers"=w370:refnum<k24>)  [unwired: 1 in, 2 out]
        n150 = invoke class="List`1[[GMap.NET.PointLatLng, G" method="Clear"(reference=w365) -> (reference out=w364:refnum<k24>)  [unwired: 2 in, 2 out]
        n151 = invoke class="ObservableCollectionThreadSafe`" method="Clear"(reference=w370) -> ()  [unwired: 2 in, 3 out]
        n152 = Bundle By Name(cluster=w369, "RefPointsCollPoly"=w364, "arrPointKeyWordOrID"=string[] [], "arrLatLngPoly"=dbl[][] [] ("arrLatLngActv")) -> (w368:T13)
      }
      frame "Error" {
      }
      frame "Exit" {
        n153 = global write "Global Var.vi" "Exit GPS"(TRUE ("EXIT-GPS")) -> ()
      }
    }
    n154 = call "Map Control.vi"("Error"=w224, "Q-IN"=w216, "QFNs"=w218, "Enum"=w217) -> ()  [unwired: 12 in]
  }
  "Map Error" <- w38
  n155 = VISA Close(VISA resource name=w53, error in (no error)=w52) -> (error out=w62:errorcluster)
  n156 = call <vilib>:"Simple Error Handler.vi"("error in (no error)"=w62) -> ()  [unwired: 1 in, 8 out]
  n157 = Unbundle By Name(w37) -> ("dotNetGMap"=w33:refnum<k24>, "VIRef"=w36:refnum<vi>)
  n158 = Release Queue(queue=w30, force destroy? (F)=TRUE) -> ()  [unwired: 1 in, 3 out]
  n159 = invoke class="VI" method="FP.Close"(reference=w36) -> (reference out=w34:refnum<vi>)  [unwired: 2 in, 2 out]
  n160 = Close Reference(reference=w33) -> ()  [unwired: 1 in, 1 out]
  n161 = Close Reference(reference=w34) -> ()  [unwired: 1 in, 1 out]
  "MessageType" <- NMEA_Type."None" ("MessageType")
